vi "OP500ZP_GlobalVariables.vi"() -> ()   [LabVIEW 2020]
uses:
  CheminDeBase.vi
  <vilib>/Utility/config.llb/Read Key (Double).vi
  OP500ZP_VGConf.vi
  <vilib>/Utility/config.llb/Read Key (String).vi
  <vilib>/Utility/config.llb/NI_LVConfig.lvlib
panel:
  out "error out 2":errorcluster caption="error out"
  out "error out":errorcluster
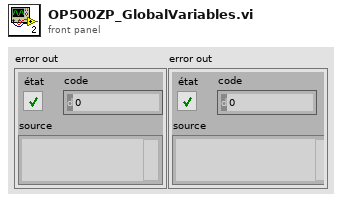
[diagram p1: front panel]
types:
  T1 = typedef "NI_LVConfig.lvlib/Config Data RefNum.ctl" = refnum<k1>
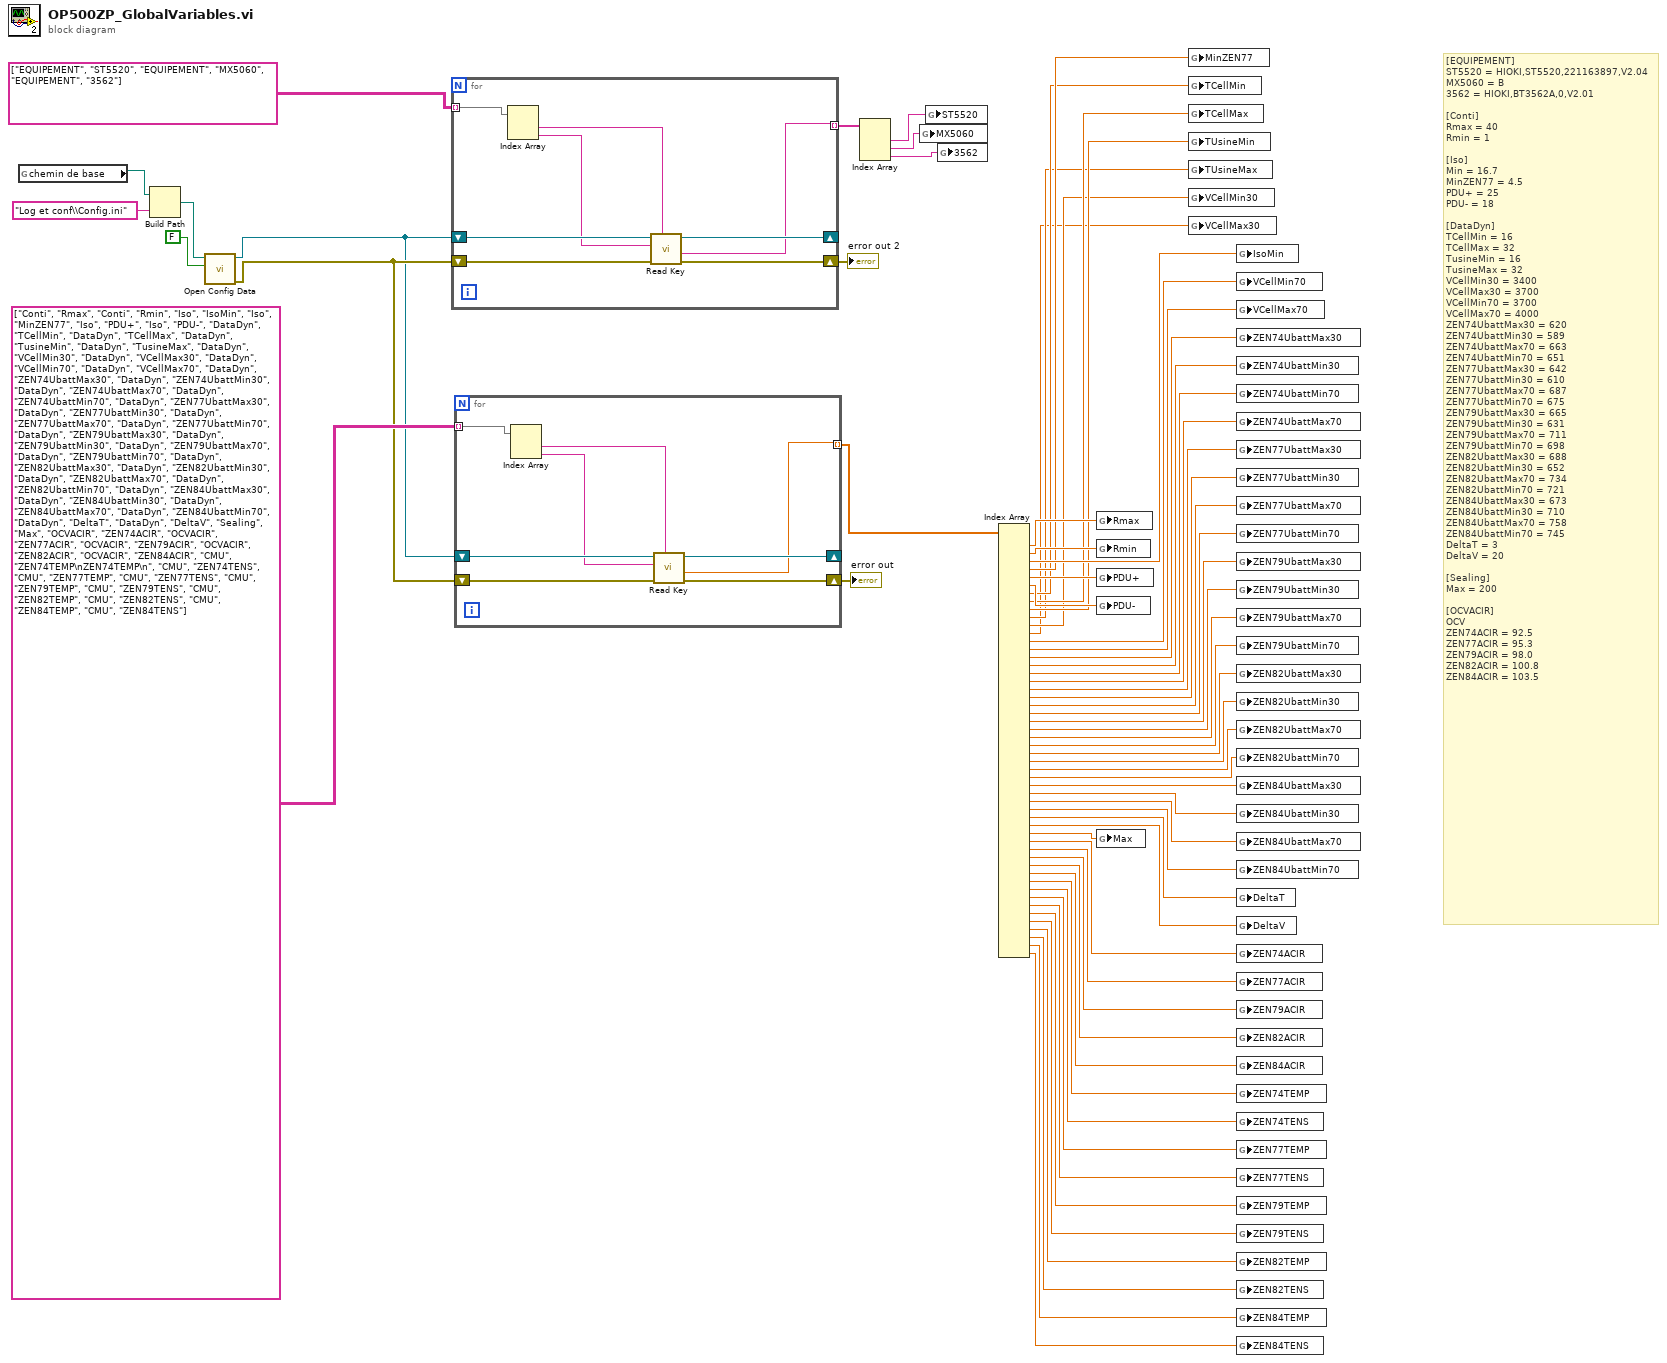
[diagram p0: block diagram]
diagram:
  # "[EQUIPEMENT]\nST5520 = HIOKI,ST5520,221163897,V2.04\t\nMX5060 = B\n3562 = HIOKI,BT3562A,0,V2.01\n\n[Conti]\nRmax = 40\nRmin = 1\n\n[Iso]\nMin = 16.7\nMinZEN77 = 4.5\nPDU+ = 25\nPDU- = 18\n\n[DataDyn]\nTCellMin = 16\nTCellMax = 32\nTusineMin = 16\nTusineMax = 32\nVCellMin30 = 3400\nVCellMax30 = 3700\nVCellMin70 = 3700\nVCellMax70 = 4000\nZEN74UbattMax30 = 620\nZEN74UbattMin30 = 589\nZEN74UbattMax70 = 663\nZEN74UbattMin70 = 651\nZEN77UbattMax30 = 642\nZEN77UbattMin30 = 610\nZEN77UbattMax70 = 687\nZEN77UbattMin70 = 675\nZEN79UbattMax30 = 665\nZEN79UbattMin30 = 631\nZEN79UbattMax70 = 711\nZEN79UbattMin70 = 698\nZEN82UbattMax30 = 688\nZEN82UbattMin30 = 652\nZEN82UbattMax70 = 734\nZEN82UbattMin70 = 721\nZEN84UbattMax30 = 673\nZEN84UbattMin30 = 710\nZEN84UbattMax70 = 758\nZEN84UbattMin70 = 745\nDeltaT = 3\nDeltaV = 20\n\n[Sealing]\nMax = 200\n\n[OCVACIR]\nOCV\nZEN74ACIR = 92.5\nZEN77ACIR = 95.3\nZEN79ACIR = 98.0\nZEN82ACIR = 100.8\nZEN84ACIR = 103.5"
  n1 = global read "CheminDeBase.vi" "chemin de base"() -> (w16:path)
  n2 = Build Path(base path=w16, name or relative path="Log et conf\\Config.ini") -> (appended path=w66:path)
  n3 = call <vilib>:"Open Config Data.vi"("create file if necessary (T)"=FALSE, "configuration file path"=w66) -> ("error out"=w20:errorcluster, "refnum"=w19:T1)  [unwired: 7 in, 1 out]
  n4 = for {
    tunnel: string[][] [["EQUIPEMENT", "ST5520"], ["EQUIPEMENT", "MX5060"], ["EQUIPEMENT", "3562"]] -> [w72] mode=indexing
    shift-right: [w73] -> w17
    shift-left: w20 -> [w75]
    shift-right: [w69] -> _
    shift-left: w19 -> [w74]
    tunnel: [w68] -> w63 mode=indexing
    n5 = Index Array(array=w72) -> (element #1=w71:string, element #2=w70:string)  [unwired: 2 in]
    n6 = call-poly <vilib>:"Read Key.vi"("section"=w71, "error in (no error)"=w75, "key"=w70, "refnum"=w74) -> ("error out"=w73:errorcluster, "value"=w68:string, "refnum out"=w69:T1)  [unwired: 4 in, 1 out]
  }
  "error out 2" <- w17
  n7 = for {
    tunnel: string[][] [["Conti", "Rmax"], ["Conti", "Rmin"], ["Iso", "IsoMin"], ["Iso", "MinZEN77"], ["Iso", "PDU+"], ["Iso", "PDU-"], ["DataDyn", "TCellMin"], ["DataDyn", "TCellMax"], ["DataDyn", "TusineMin"], ["DataDyn", "TusineMax"], ["DataDyn", "VCellMin30"], ["DataDyn", "VCellMax30"], ["DataDyn", "VCellMin70"], ["DataDyn", "VCellMax70"], ["DataDyn", "ZEN74UbattMax30"], ["DataDyn", "ZEN74UbattMin30"], ["DataDyn", "ZEN74UbattMax70"], ["DataDyn", "ZEN74UbattMin70"], ["DataDyn", "ZEN77UbattMax30"], ["DataDyn", "ZEN77UbattMin30"], ["DataDyn", "ZEN77UbattMax70"], ["DataDyn", "ZEN77UbattMin70"], ["DataDyn", "ZEN79UbattMax30"], ["DataDyn", "ZEN79UbattMin30"], ["DataDyn", "ZEN79UbattMax70"], ["DataDyn", "ZEN79UbattMin70"], ["DataDyn", "ZEN82UbattMax30"], ["DataDyn", "ZEN82UbattMin30"], ["DataDyn", "ZEN82UbattMax70"], ["DataDyn", "ZEN82UbattMin70"], ["DataDyn", "ZEN84UbattMax30"], ["DataDyn", "ZEN84UbattMin30"], ["DataDyn", "ZEN84UbattMax70"], ["DataDyn", "ZEN84UbattMin70"], ["DataDyn", "DeltaT"], ["DataDyn", "DeltaV"], ["Sealing", "Max"], ["OCVACIR", "ZEN74ACIR"], ["OCVACIR", "ZEN77ACIR"], ["OCVACIR", "ZEN79ACIR"], ["OCVACIR", "ZEN82ACIR"], ["OCVACIR", "ZEN84ACIR"], ["CMU", "ZEN74TEMP\nZEN74TEMP\n"], ["CMU", "ZEN74TENS"], ["CMU", "ZEN77TEMP"], ["CMU", "ZEN77TENS"], ["CMU", "ZEN79TEMP"], ["CMU", "ZEN79TENS"], ["CMU", "ZEN82TEMP"], ["CMU", "ZEN82TENS"], ["CMU", "ZEN84TEMP"], ["CMU", "ZEN84TENS"]] -> [w80] mode=indexing
    shift-right: [w81] -> w18
    shift-left: w20 -> [w83]
    shift-right: [w77] -> _
    shift-left: w19 -> [w82]
    tunnel: [w76] -> w58 mode=indexing
    n8 = Index Array(array=w80) -> (element #1=w79:string, element #2=w78:string)  [unwired: 2 in]
    n9 = call-poly <vilib>:"Read Key.vi"("section"=w79, "error in (no error)"=w83, "key"=w78, "refnum"=w82) -> ("error out"=w81:errorcluster, "value"=w76:dbl, "refnum out"=w77:T1)  [unwired: 4 in, 1 out]
  }
  "error out" <- w18
  n10 = Index Array(array=w63) -> (element #1=w62:string, element #2=w61:string, element #3=w60:string)  [unwired: 3 in]
  n11 = global write "OP500ZP_VGConf.vi" "MX5060"(w61) -> ()
  n12 = global write "OP500ZP_VGConf.vi" "ST5520"(w62) -> ()
  n13 = global write "OP500ZP_VGConf.vi" "3562"(w60) -> ()
  n14 = Index Array(array=w58) -> (element #1=w57:dbl, element #2=w56:dbl, element #3=w55:dbl, element #4=w54:dbl, element #5=w53:dbl, element #6=w52:dbl, element #7=w51:dbl, element #8=w50:dbl, element #9=w49:dbl, element #10=w48:dbl, element #11=w47:dbl, element #12=w46:dbl, element #13=w45:dbl, element #14=w44:dbl, element #15=w43:dbl, element #16=w42:dbl, element #17=w41:dbl, element #18=w40:dbl, element #19=w39:dbl, element #20=w38:dbl, element #21=w37:dbl, element #22=w36:dbl, element #23=w35:dbl, element #24=w34:dbl, element #25=w33:dbl, element #26=w32:dbl, element #27=w31:dbl, element #28=w30:dbl, element #29=w29:dbl, element #30=w28:dbl, element #31=w27:dbl, element #32=w26:dbl, element #33=w25:dbl, element #34=w24:dbl, element #35=w23:dbl, element #36=w22:dbl, element #37=w21:dbl, element #38=w15:dbl, element #39=w14:dbl, element #40=w13:dbl, element #41=w12:dbl, element #42=w11:dbl, element #43=w10:dbl, element #44=w9:dbl, element #45=w8:dbl, element #46=w7:dbl, element #47=w6:dbl, element #48=w5:dbl, element #49=w4:dbl, element #50=w3:dbl, element #51=w2:dbl, element #52=w1:dbl)  [unwired: 52 in]
  n15 = global write "OP500ZP_VGConf.vi" "Rmax"(w57) -> ()
  n16 = global write "OP500ZP_VGConf.vi" "Rmin"(w56) -> ()
  n17 = global write "OP500ZP_VGConf.vi" "PDU+"(w53) -> ()
  n18 = global write "OP500ZP_VGConf.vi" "PDU-"(w52) -> ()
  n19 = global write "OP500ZP_VGConf.vi" "Max"(w21) -> ()
  n20 = global write "OP500ZP_VGConf.vi" "MinZEN77"(w54) -> ()
  n21 = global write "OP500ZP_VGConf.vi" "TCellMin"(w51) -> ()
  n22 = global write "OP500ZP_VGConf.vi" "TCellMax"(w50) -> ()
  n23 = global write "OP500ZP_VGConf.vi" "TUsineMin"(w49) -> ()
  n24 = global write "OP500ZP_VGConf.vi" "TUsineMax"(w48) -> ()
  n25 = global write "OP500ZP_VGConf.vi" "VCellMin30"(w47) -> ()
  n26 = global write "OP500ZP_VGConf.vi" "VCellMax30"(w46) -> ()
  n27 = global write "OP500ZP_VGConf.vi" "IsoMin"(w55) -> ()
  n28 = global write "OP500ZP_VGConf.vi" "VCellMin70"(w45) -> ()
  n29 = global write "OP500ZP_VGConf.vi" "VCellMax70"(w44) -> ()
  n30 = global write "OP500ZP_VGConf.vi" "ZEN74UbattMax30"(w43) -> ()
  n31 = global write "OP500ZP_VGConf.vi" "ZEN74UbattMin30"(w42) -> ()
  n32 = global write "OP500ZP_VGConf.vi" "ZEN74UbattMin70"(w41) -> ()
  n33 = global write "OP500ZP_VGConf.vi" "ZEN74UbattMax70"(w40) -> ()
  n34 = global write "OP500ZP_VGConf.vi" "ZEN77UbattMax30"(w39) -> ()
  n35 = global write "OP500ZP_VGConf.vi" "ZEN77UbattMin30"(w38) -> ()
  n36 = global write "OP500ZP_VGConf.vi" "ZEN77UbattMax70"(w37) -> ()
  n37 = global write "OP500ZP_VGConf.vi" "ZEN77UbattMin70"(w36) -> ()
  n38 = global write "OP500ZP_VGConf.vi" "ZEN79UbattMax30"(w35) -> ()
  n39 = global write "OP500ZP_VGConf.vi" "ZEN79UbattMin30"(w34) -> ()
  n40 = global write "OP500ZP_VGConf.vi" "ZEN79UbattMax70"(w33) -> ()
  n41 = global write "OP500ZP_VGConf.vi" "ZEN79UbattMin70"(w32) -> ()
  n42 = global write "OP500ZP_VGConf.vi" "ZEN82UbattMax30"(w31) -> ()
  n43 = global write "OP500ZP_VGConf.vi" "ZEN82UbattMin30"(w30) -> ()
  n44 = global write "OP500ZP_VGConf.vi" "ZEN82UbattMax70"(w29) -> ()
  n45 = global write "OP500ZP_VGConf.vi" "ZEN82UbattMin70"(w28) -> ()
  n46 = global write "OP500ZP_VGConf.vi" "ZEN84UbattMax30"(w27) -> ()
  n47 = global write "OP500ZP_VGConf.vi" "ZEN84UbattMin30"(w26) -> ()
  n48 = global write "OP500ZP_VGConf.vi" "ZEN84UbattMax70"(w25) -> ()
  n49 = global write "OP500ZP_VGConf.vi" "ZEN84UbattMin70"(w24) -> ()
  n50 = global write "OP500ZP_VGConf.vi" "DeltaT"(w23) -> ()
  n51 = global write "OP500ZP_VGConf.vi" "DeltaV"(w22) -> ()
  n52 = global write "OP500ZP_VGConf.vi" "ZEN74ACIR"(w15) -> ()
  n53 = global write "OP500ZP_VGConf.vi" "ZEN77ACIR"(w14) -> ()
  n54 = global write "OP500ZP_VGConf.vi" "ZEN79ACIR"(w13) -> ()
  n55 = global write "OP500ZP_VGConf.vi" "ZEN82ACIR"(w12) -> ()
  n56 = global write "OP500ZP_VGConf.vi" "ZEN84ACIR"(w11) -> ()
  n57 = global write "OP500ZP_VGConf.vi" "ZEN74TEMP"(w10) -> ()
  n58 = global write "OP500ZP_VGConf.vi" "ZEN74TENS"(w9) -> ()
  n59 = global write "OP500ZP_VGConf.vi" "ZEN77TEMP"(w8) -> ()
  n60 = global write "OP500ZP_VGConf.vi" "ZEN77TENS"(w7) -> ()
  n61 = global write "OP500ZP_VGConf.vi" "ZEN79TEMP"(w6) -> ()
  n62 = global write "OP500ZP_VGConf.vi" "ZEN79TENS"(w5) -> ()
  n63 = global write "OP500ZP_VGConf.vi" "ZEN82TEMP"(w4) -> ()
  n64 = global write "OP500ZP_VGConf.vi" "ZEN82TENS"(w3) -> ()
  n65 = global write "OP500ZP_VGConf.vi" "ZEN84TEMP"(w2) -> ()
  n66 = global write "OP500ZP_VGConf.vi" "ZEN84TENS"(w1) -> ()
